vi "set_params.vi"(8 "error in (no error)":errorcluster caption="entrée d'erreur (pas d'erreur)", 11 "KernelPCA.lvclass 2":refnum<class "KernelPCA.lvclass">) -> (0 "error out":errorcluster caption="sortie d'erreur", 3 "KernelPCA.lvclass":refnum<class "KernelPCA.lvclass">)   [LabVIEW 2020, in "KernelPCA.lvclass"]
uses:
  KernelPCA.lvclass
  KernelPCA.lvclass/KernelPCA.ctl
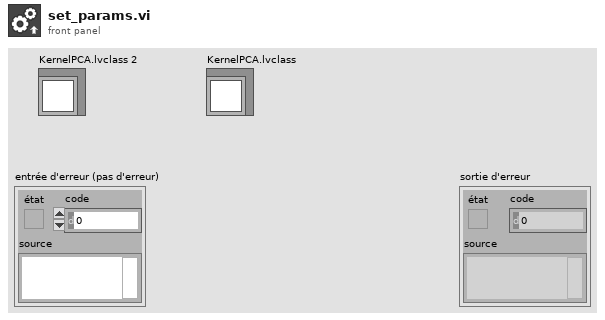
[diagram p1: front panel]
types:
  T1 = typedef "kernel_pca_params.ctl" = cluster{"n_components":cluster{"n_components_type":string, "n_components_int":dbl}, "kernel":string, "gamma":cluster{"gamma_float":dbl, "gamma_type":string}, "degree":dbl, "coef0":dbl, "alpha":dbl, "fit_inverse_transform":bool, "eigen_solver":string, "tol":dbl, "max_iter":cluster{"max_iter_type":string, "max_iter_int":dbl}, "remove_zero_eig":bool, "random_state":dbl, "copy_X":bool, "n_jobs":dbl}
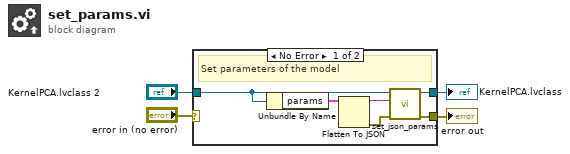
[diagram p0: block diagram]
diagram:
  n1 = case shown="No Error" "error in (no error)" {
    selector: "error in (no error)" -> [_ w12]
    tunnel: [w7 w12] -> w3
    tunnel: [w8 w11] -> w1
    tunnel: "KernelPCA.lvclass 2" -> [w5 w11]
    frame No Error {
      # "Set parameters of the model"
      n2 = Unbundle By Name(w5) -> ("params"=w10:T1)
      n3 = Flatten To JSON(anything=w10) -> (JSON string=w9:string, 11:w6:errorcluster)  [unwired: 2 in]
      n4 = call-dynamic "set_json_params.vi"("error in (no error)"=w6, "params"=w9, "Model en entrée"=w5) -> ("error out"=w7:errorcluster, "Model en sortie"=w8:refnum<class "KernelPCA.lvclass">)  [unwired: 7 in]
    }
    frame Error {
    }
  }
  "error out" <- w3
  "KernelPCA.lvclass" <- w1
